vi "projekt.vi"() -> ()   [LabVIEW 2023]
doc: "Use this template to build a standard state machine design pattern. Each state executes code and determines which state to transition to. Contrast this design pattern with the User Interface Event Handler pattern, in which code executes in response to user actions. Contrast this design pattern also with the Queued Message Handler pattern, in which each message handling code can queue zero or more new messages.\nNote: This template does not contain the most recent programming guidelines recommended by National Instruments. For a complete, project-based implementation of the Standard State Machine pattern, use the Create Project dialog box instead of this template."
uses:
  projekt.ctl
  <vilib>/DAQmx/read.llb/DAQmx Read (Analog DBL 1Chan 1Samp).vi
  <vilib>/DAQmx/read.llb/DAQmx Read (Digital 1D Bool 1Chan 1Samp).vi
  <vilib>/DAQmx/write.llb/DAQmx Write (Digital 1D Bool 1Chan 1Samp).vi
  <vilib>/DAQmx/create/channels.llb/DAQmx Create Channel (AI-Voltage-Basic).vi
  <vilib>/DAQmx/create/channels.llb/DAQmx Create Channel (DI-Digital Input).vi
  <vilib>/DAQmx/create/channels.llb/DAQmx Create Channel (DO-Digital Output).vi
  <vilib>/Utility/file.llb/Read Delimited Spreadsheet (DBL).vi
  <vilib>/DAQmx/miscellaneous.llb/DAQmx Fill In Error Info.vi
  <vilib>/Utility/file.llb/Write Delimited Spreadsheet (DBL).vi
panel:
  out "TRYB":string="USTAWIENIA"
  out "wynik":i32
  out "punkty za ruch":i32=6
  out "czas wyswietlania":u32=250
  out "check index":i32
  out "now click":u32
  in  "time options":u32[](array[numeric])=[250, 500, 750, 1000, 1250, 1500]
  out "TOP WYNIKI":string="4\n4\r\n"
  out "?":string
  out "check result":bool
  in  "file path (dialog if empty)":path
  out "sekwencja":string="2\r\n"
  out "level":i32
  in  "stop":bool
  in  "Diody wynik":tag="Dev2/port0/line3:5"
  in  "Diody gorne":tag="Dev2/port0/line0:2"
  in  "Przyciski":tag="Dev2/port1/line0:2"
  in  "Pokretlo":tag="Dev2/ai1"
  # "TRYB USTAWIENIA:\nMozesz regulowac czas wyswietlania elementu sekwencji, wplywa to na liczbe punktow przyznawana za kazdy poprawny ruch.\nAby rozpoczac gre kliknij zielony guzik.\n\nTRYB GRY:\nPo wyswietleniu sekwencji na gornych diodach odwzoruj ja na guzikach.\n\nPo przegranej mozesz ponownie rozpoczac gre zielonym guzikiem!"
  # "4 green 2 yellow 1 red"
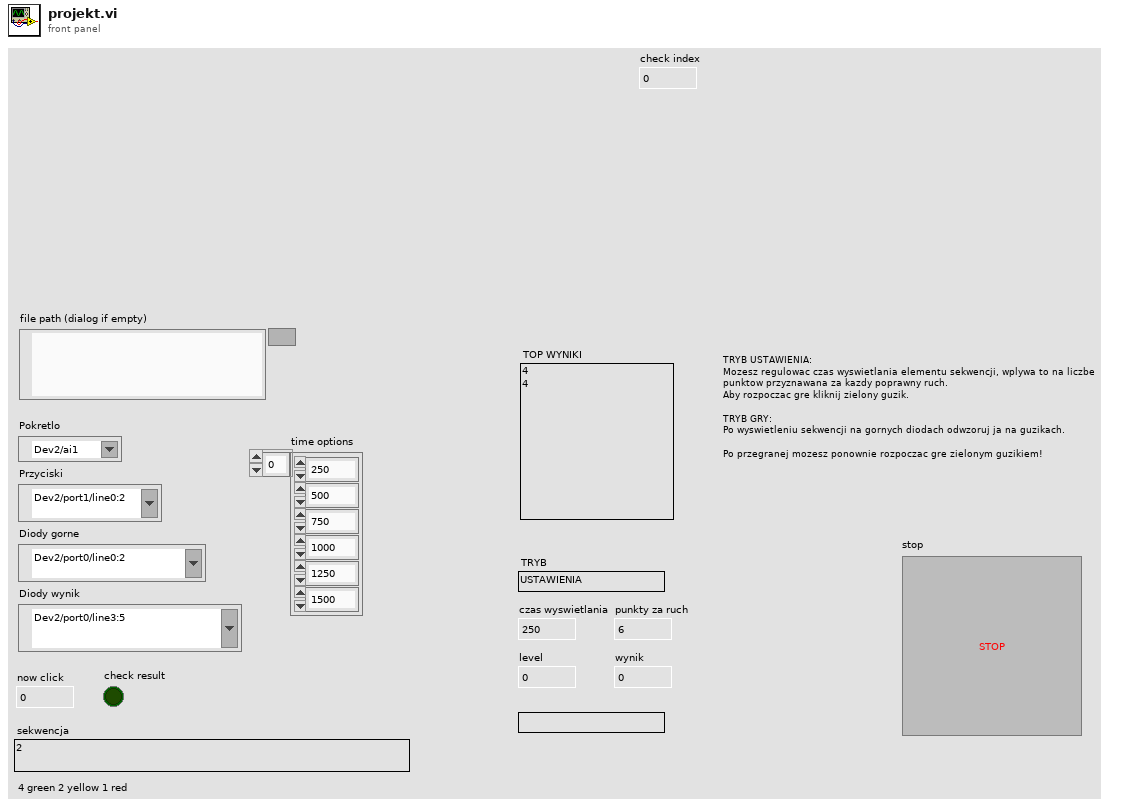
[diagram p1: front panel]
types:
  T1 = typedef "projekt.ctl" = enum16{"Initialize", "Start", "Add element", "Display ", "Check", "Game over", "Game result", "High score", "Stop"}
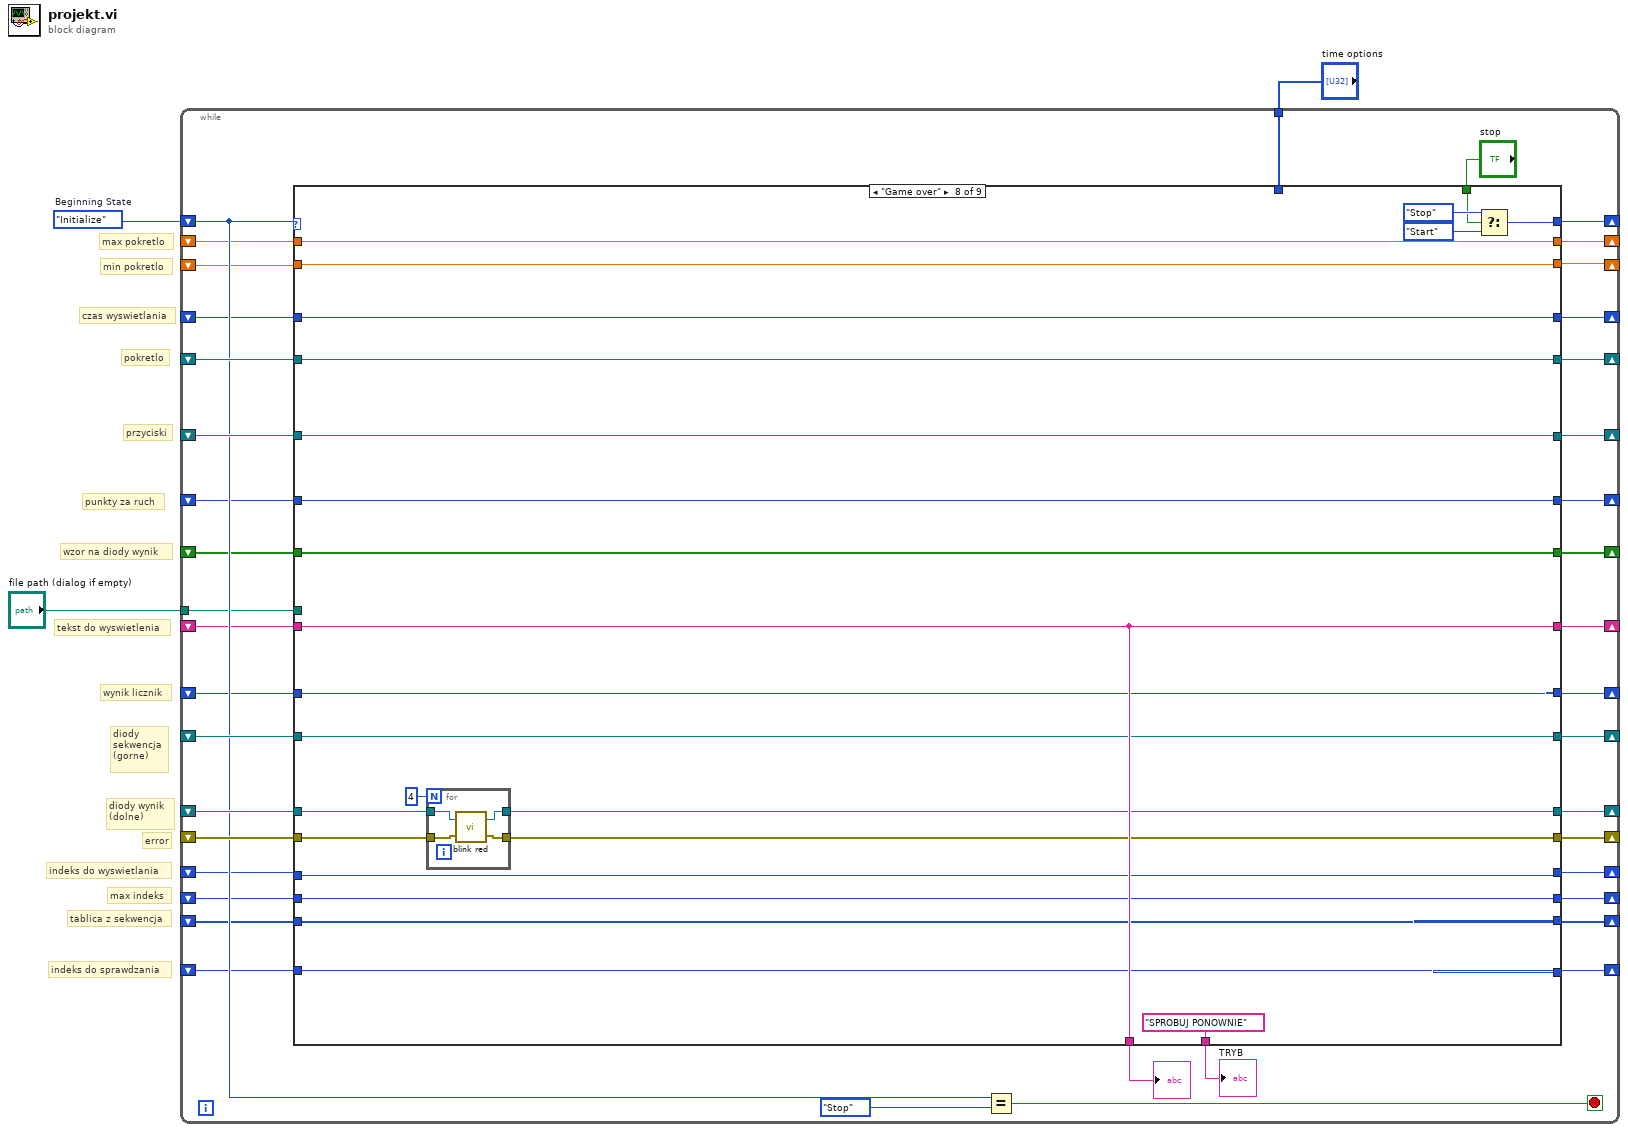
[diagram p0: block diagram]
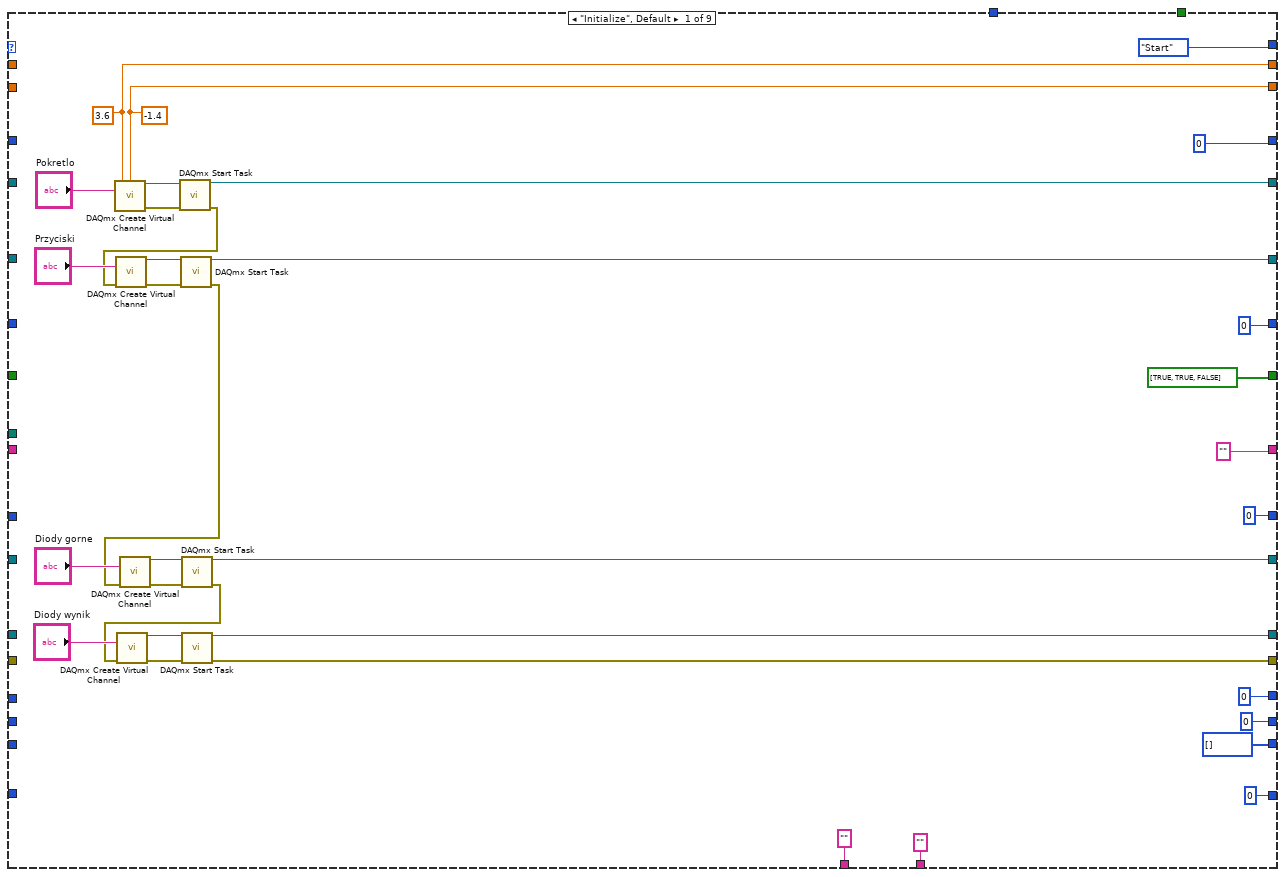
[diagram p2: hidden frame]
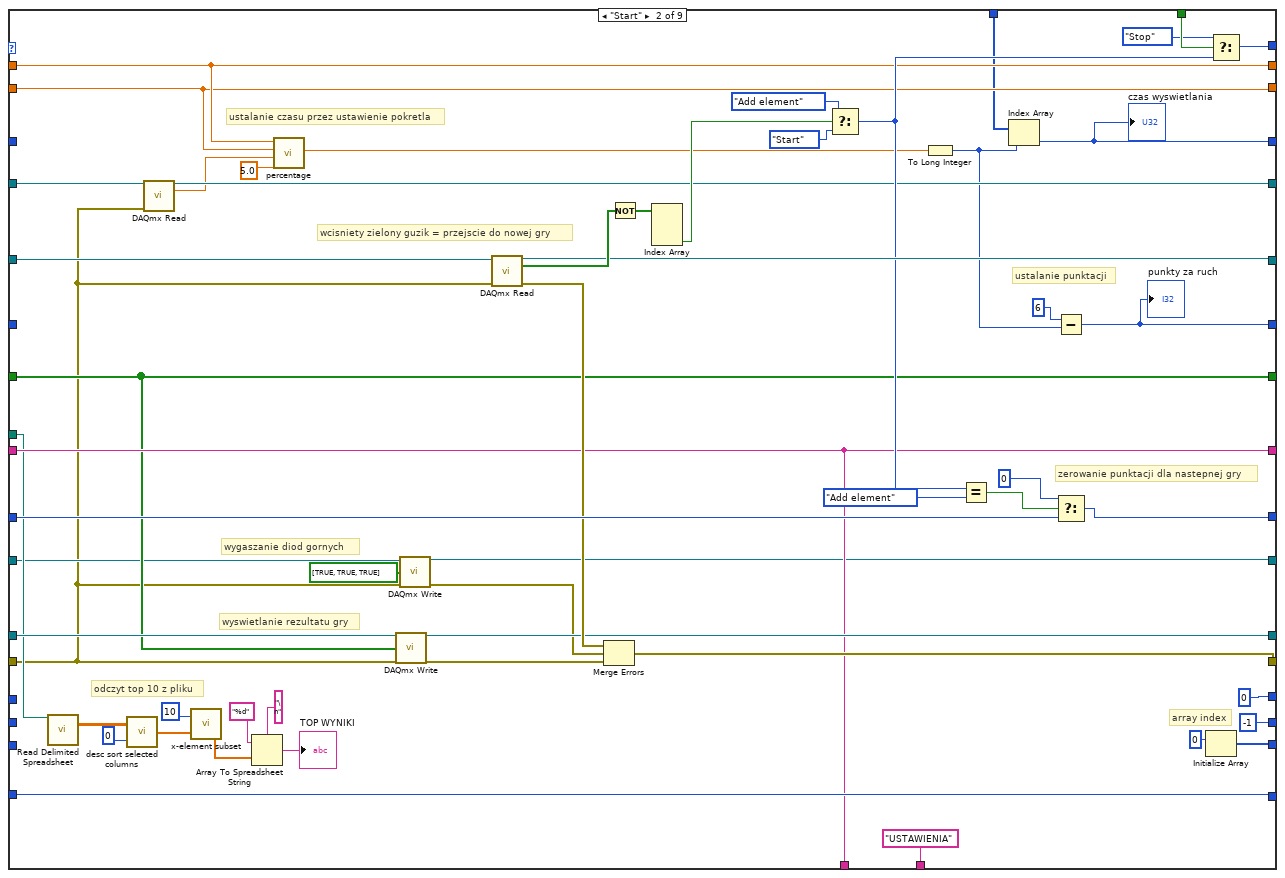
[diagram p3: hidden frame]
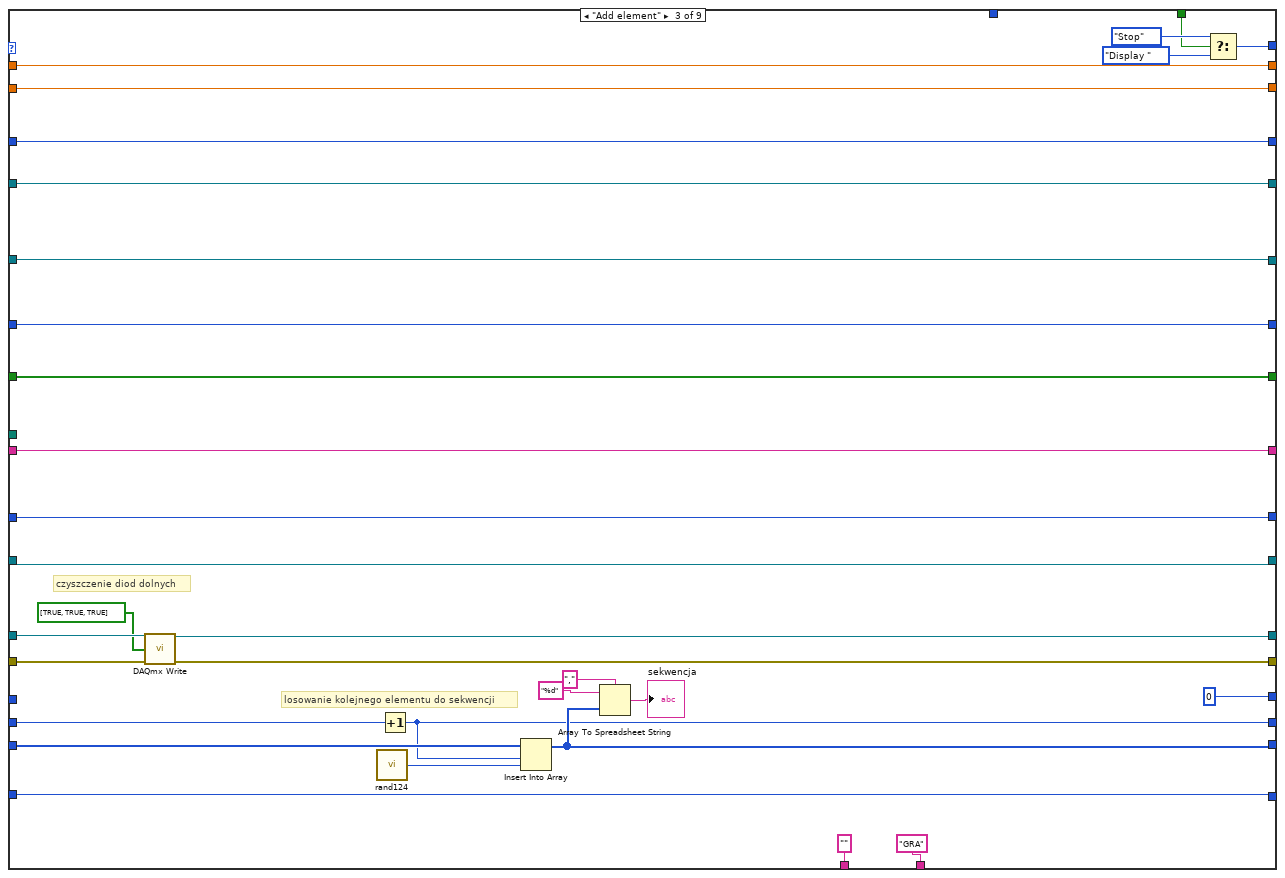
[diagram p4: hidden frame]
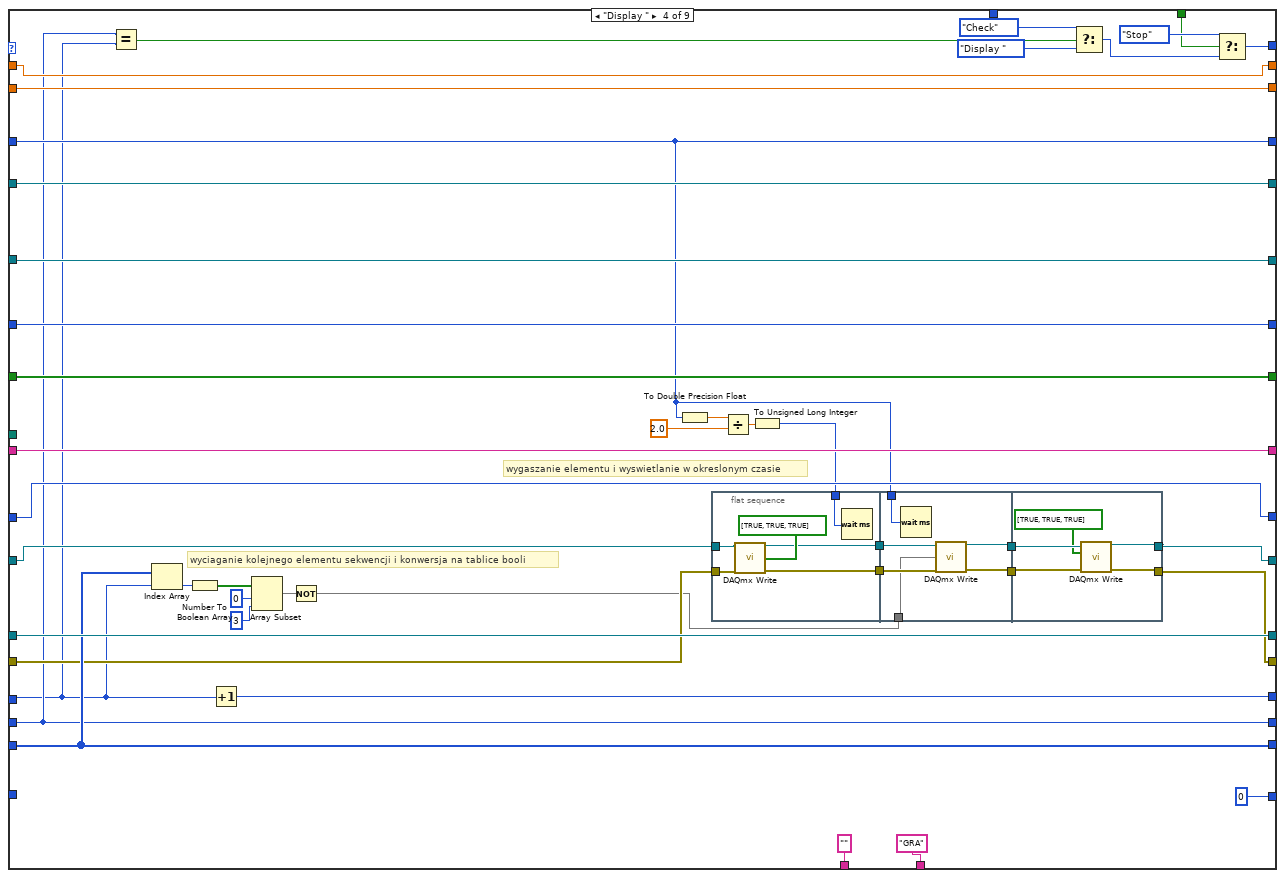
[diagram p5: hidden frame]
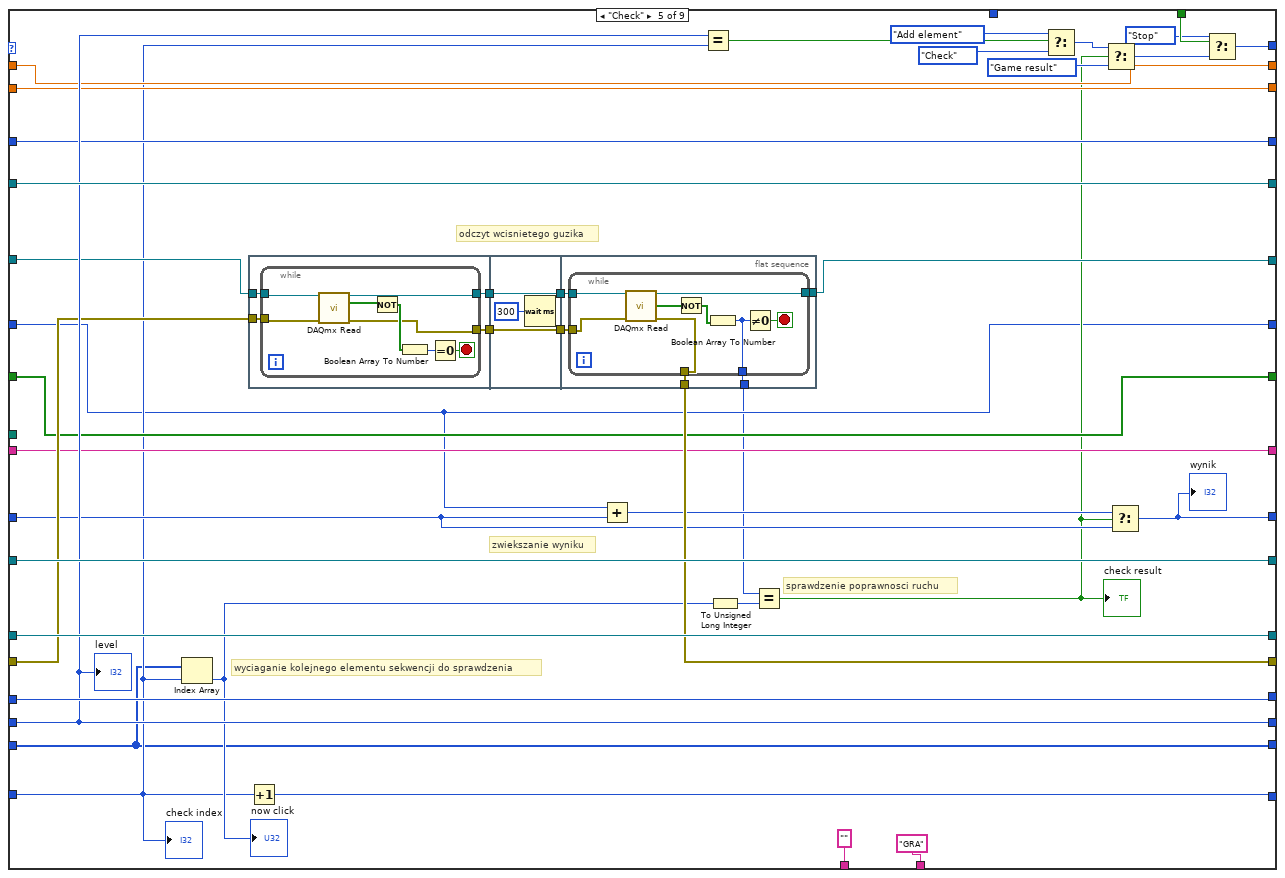
[diagram p6: hidden frame]
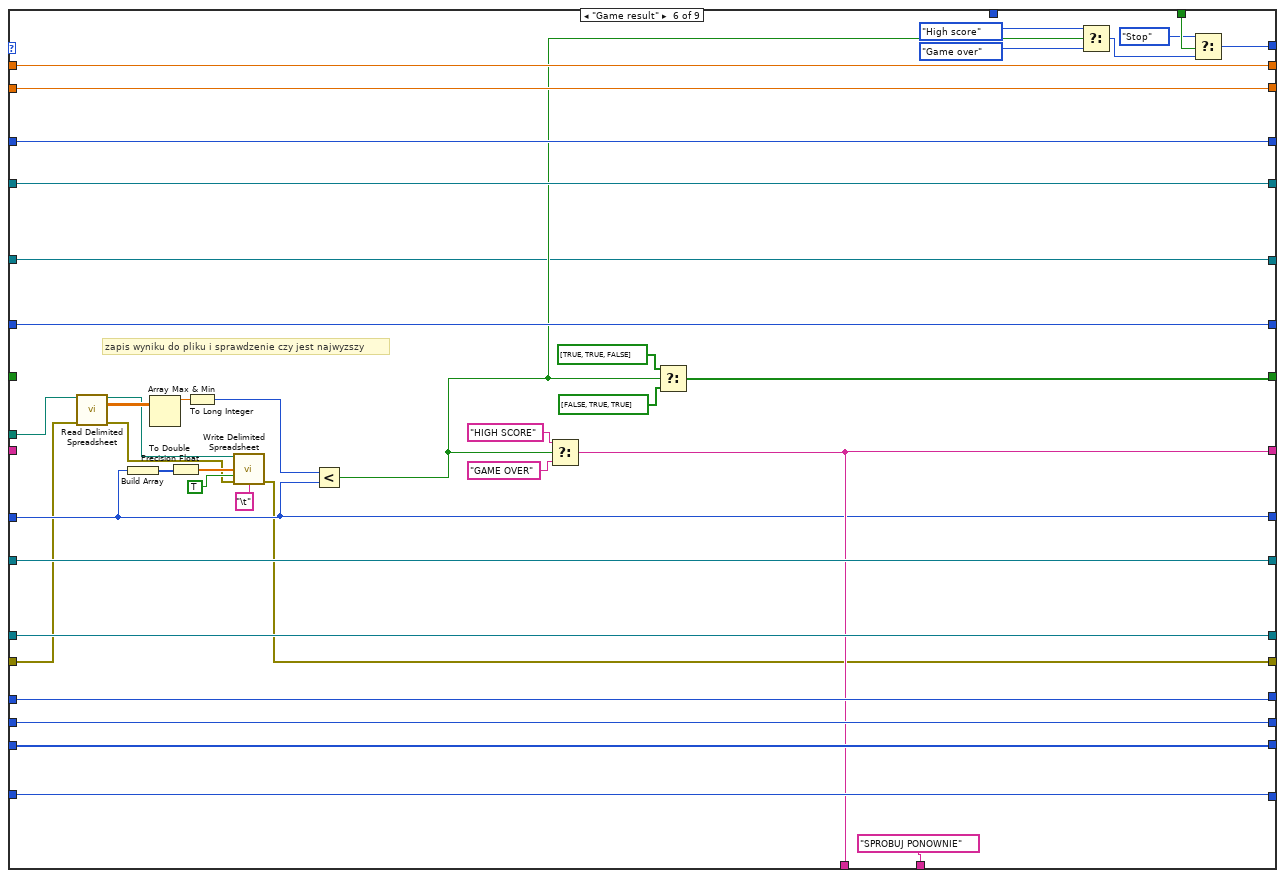
[diagram p7: hidden frame]
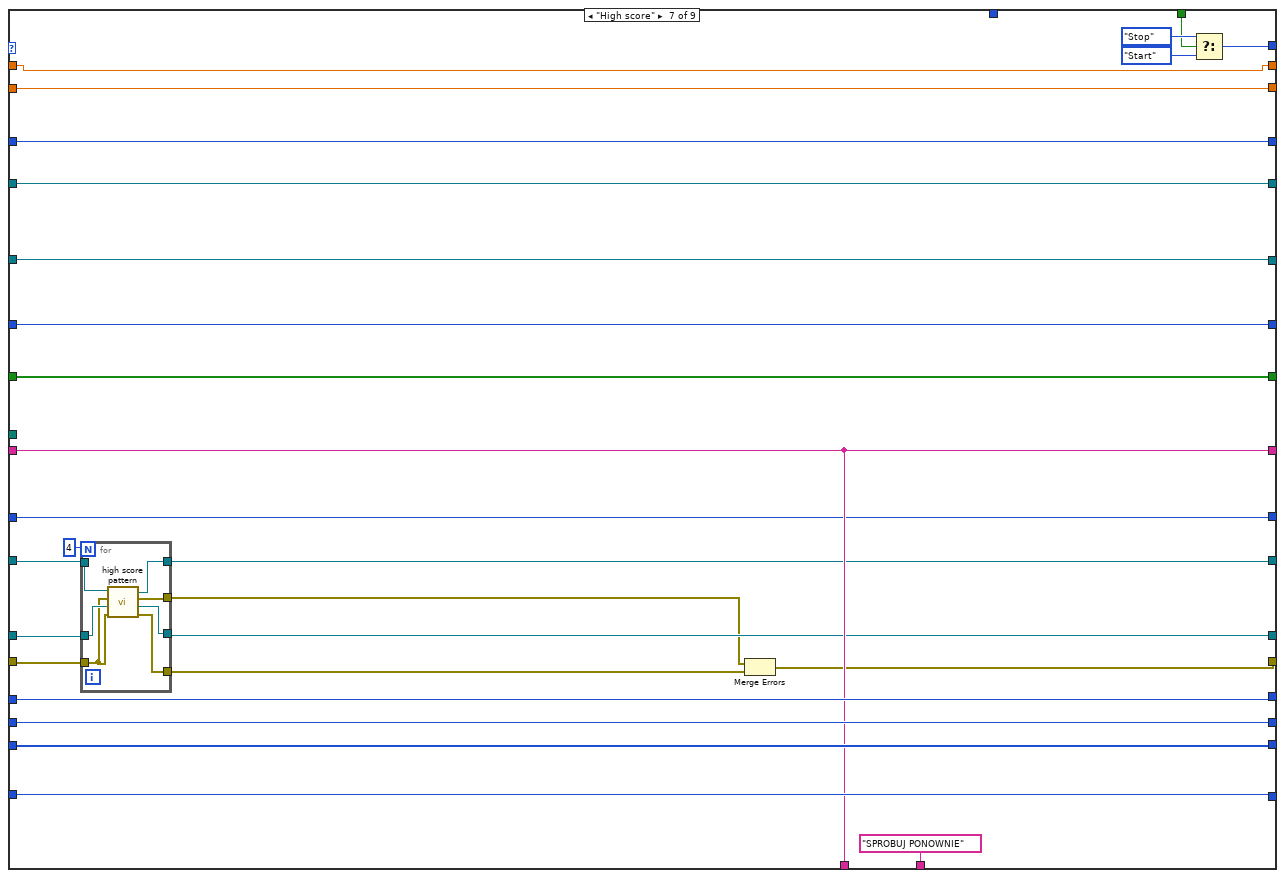
[diagram p8: hidden frame]
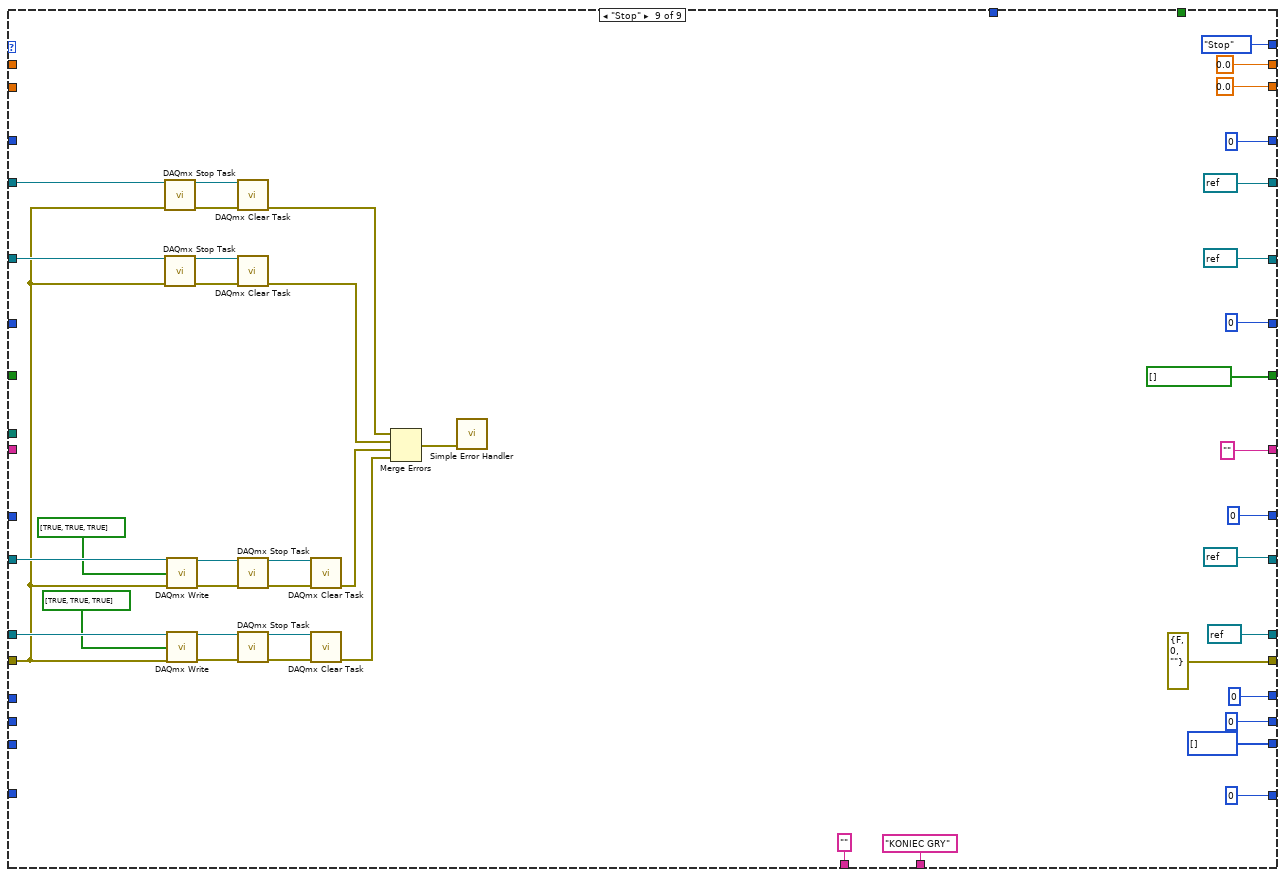
[diagram p9: hidden frame]
diagram:
  w3 = projekt."Initialize"  # Beginning State
  # "tekst do wyswietlenia"
  # "punkty za ruch"
  # "czas wyswietlania"
  # "max pokretlo"
  # "min pokretlo"
  # "wzor na diody wynik"
  # "wynik licznik"
  # "indeks do sprawdzania"
  # "tablica z sekwencja"
  # "max indeks"
  # "indeks do wyswietlania"
  # "error"
  # "diody wynik\n(dolne)"
  # "diody \nsekwencja\n(gorne)"
  # "przyciski"
  # "pokretlo"
  n1 = while {
    shift-right: [w42] -> _
    shift-left: w3 -> [w30]
    shift-right: [w34] -> _
    shift-left: _ -> [w35]
    shift-right: [w41] -> _
    shift-left: _ -> [w38]
    shift-right: [w33] -> _
    shift-left: _ -> [w39]
    shift-right: [w32] -> _
    shift-left: _ -> [w36]
    shift-right: [w40] -> _
    shift-left: _ -> [w37]
    shift-right: [w24] -> _
    shift-left: _ -> [w27]
    shift-right: [w29] -> _
    shift-left: _ -> [w28]
    shift-right: [w26] -> _
    shift-left: _ -> [w25]
    shift-right: [w23] -> _
    shift-left: _ -> [w22]
    shift-right: [w19] -> _
    shift-left: _ -> [w20]
    shift-right: [w18] -> _
    shift-left: _ -> [w17]
    shift-right: [w16] -> _
    shift-left: _ -> [w15]
    shift-right: [w14] -> _
    shift-left: _ -> [w11]
    shift-right: [w13] -> _
    shift-left: _ -> [w12]
    shift-right: [w10] -> _
    shift-left: _ -> [w9]
    tunnel: "file path (dialog if empty)" -> [w8]
    tunnel: "time options" -> [w7]
    shift-right: [w6] -> _
    shift-left: _ -> [w5]
    stop <- w44 stop-if-true
    n2 = case shown="\"Game over\"" w30 {
      tunnel: [projekt."Start" w127 w159 w199 w236 w324 w354 w385 projekt."Stop" ("Next State")] -> w42
      tunnel: [w66 w112 w146 w206 w261 w329 w335 w369 refnum<k21> refnum ("task out")] -> w41
      tunnel: [w65 w130 w163 w205 w254 w303 w349 w380 refnum<k21> refnum ("task out")] -> w40
      tunnel: w39 -> [_ w85 w162 w195 w262 w330 w337 w375 w418]
      tunnel: w38 -> [_ w115 w147 w206 w261 w329 w338 w370 w415]
      tunnel: w37 -> [_ w133 w163 w205 w256 w303 w349 w380 w428]
      tunnel: w36 -> [_ w109 w164 w204 w263 w322 w350 w381 w421]
      tunnel: w35 -> [_ w83 w145 w196 w255 w294 w339 w368 w404]
      tunnel: [w64 w113 w144 w192 w253 w295 w341 w367 errorcluster {"status"=FALSE, "code"=0, "source"=""} ("error out")] -> w34
      tunnel: [w63 w84 w162 w189 w262 w330 w333 w375 refnum<k21> refnum ("task out")] -> w33
      tunnel: [w62 w108 w164 w204 w263 w322 w350 w381 refnum<k21> refnum ("task out")] -> w32
      tunnel: "stop" -> [_ w129 w158 w200 w239 w325 w355 w386 _]
      tunnel: [u32[] [] w123 w154 w202 w225 w327 w344 w372 u32[] []] -> w24
      tunnel: w27 -> [_ _ w161 w202 w225 w327 w344 w372 _]
      tunnel: [0 -1 w139 w169 w259 w321 w345 w373 0] -> w29
      tunnel: w28 -> [_ _ w156 w169 w259 w321 w345 w373 _]
      tunnel: [0 0 0 w203 w260 w328 w346 w374 0] -> w26
      tunnel: w25 -> [_ _ _ w168 w260 w328 w346 w374 _]
      tunnel: [0 w121 w155 0 w248 w326 w343 w371 0] -> w23
      tunnel: w22 -> [_ w121 w155 _ w229 w326 w343 w371 _]
      tunnel: ["" w111 "" "" "" w311 w342 w378 ""] -> w21
      tunnel: w20 -> [_ w116 w150 w188 w232 w310 w340 w376 _]
      tunnel: [0 ("t") w117 w150 w188 w242 w310 w340 w376 0] -> w19
      tunnel: ["" w111 w148 w186 w240 w311 w342 w378 ""] -> w18
      tunnel: w17 -> [_ w111 w148 w186 w240 _ w342 w378 _]
      tunnel: [bool[] [TRUE, TRUE, FALSE] ("data") w110 w149 w187 w241 w316 w347 w377 bool[] [] ("data")] -> w16
      tunnel: w15 -> [_ w110 w149 w187 w241 _ w347 w377 _]
      tunnel: [w55 w101 w141 w184 w234 w314 w352 w383 0.0 ("minimum value")] -> w14
      tunnel: [w54 w102 w142 w185 w235 w315 w353 w384 0.0 ("maximum value")] -> w13
      tunnel: w12 -> [_ w102 w142 w185 w235 w315 w353 w384 _]
      tunnel: w11 -> [_ w101 w141 w184 w234 w314 w352 w383 _]
      tunnel: [u32 0 ("Numeric") w99 w140 w175 w233 w313 w351 w382 u32 0 ("Numeric")] -> w10
      tunnel: w9 -> [_ _ w140 w175 w233 w313 w351 w382 _]
      tunnel: w8 -> [_ w107 _ _ _ w300 _ _ _]
      tunnel: w7 -> [_ w98 _ _ _ _ _ _ _]
      tunnel: [0 w90 w137 w179 w227 w312 w348 w379 0] -> w6
      tunnel: w5 -> [_ _ w137 w179 w227 w312 w348 w379 _]
      tunnel: ["" "USTAWIENIA" "GRA" "GRA" "GRA" "SPROBUJ PONOWNIE" "SPROBUJ PONOWNIE" "SPROBUJ PONOWNIE" "KONIEC GRY"] -> w4
      frame "Initialize", Default {
        w54 = 3.6 ("maximum value")
        w55 = -1.4 ("minimum value")
        n3 = call-poly <vilib>:"DAQmx Create Virtual Channel.vi"("maximum value"=w54, "minimum value"=w55, "physical channels"="Pokretlo") -> ("task out"=w73:refnum<k21>, "error out"=w74:errorcluster)  [unwired: 11 in]
        n4 = call <vilib>:"DAQmx Start Task.vi"("task/channels in"=w73, "error in"=w74) -> ("task out"=w62:refnum<k21>, "error out"=w53:errorcluster)  [unwired: 12 in]
        n5 = call-poly <vilib>:"DAQmx Create Virtual Channel.vi"("lines"="Przyciski", "error in"=w53) -> ("task out"=w60:refnum<k21>, "error out"=w59:errorcluster)  [unwired: 12 in]
        n6 = call <vilib>:"DAQmx Start Task.vi"("task/channels in"=w60, "error in"=w59) -> ("task out"=w65:refnum<k21>, "error out"=w68:errorcluster)  [unwired: 12 in]
        n7 = call-poly <vilib>:"DAQmx Create Virtual Channel.vi"("lines"="Diody gorne", "error in"=w68) -> ("task out"=w72:refnum<k21>, "error out"=w71:errorcluster)  [unwired: 12 in]
        n8 = call <vilib>:"DAQmx Start Task.vi"("task/channels in"=w72, "error in"=w71) -> ("task out"=w63:refnum<k21>, "error out"=w67:errorcluster)  [unwired: 12 in]
        n9 = call-poly <vilib>:"DAQmx Create Virtual Channel.vi"("lines"="Diody wynik", "error in"=w67) -> ("task out"=w70:refnum<k21>, "error out"=w69:errorcluster)  [unwired: 12 in]
        n10 = call <vilib>:"DAQmx Start Task.vi"("task/channels in"=w70, "error in"=w69) -> ("task out"=w66:refnum<k21>, "error out"=w64:errorcluster)  [unwired: 12 in]
      }
      frame "Start" {
        # "zerowanie punktacji dla nastepnej gry"
        # "wyswietlanie rezultatu gry"
        # "wygaszanie diod gornych"
        # "ustalanie punktacji"
        # "wcisniety zielony guzik = przejscie do nowej gry"
        # "ustalanie czasu przez ustawienie pokretla"
        # "odczyt top 10 z pliku"
        # "array index"
        n11 = call-poly <vilib>:"Read Delimited Spreadsheet.vi"("file path (dialog if empty)"=w107) -> ("all rows"=w96:dbl[][])  [unwired: 9 in, 5 out]
        n12 = call "desc sort selected columns.vi"("disabled index (col)"=0, "all rows in"=w96) -> ("1d sorted array (desc)"=w94:dbl[])
        n13 = call-poly <vilib>:"DAQmx Read.vi"("task/channels in"=w109, "error in"=w83) -> ("task out"=w108:refnum<k21>, "data"=w103:dbl)  [unwired: 11 in, 1 out]
        n14 = call "x-element subset.vi"("input array"=w94, "x elements"=10 ("y")) -> ("array subset"=w93:dbl[])
        n15 = Array To Spreadsheet String(delimiter (Tab)="\n", array=w93, 3:"%d" ("format string")) -> (spreadsheet string=→"TOP WYNIKI":string)
        n16 = call "percentage.vi"("max range"=5.0, "data read"=w103, "minimum value"=w101, "maximum value"=w102) -> ("percentage of mac range"=w91:dbl)
        n17 = call-poly <vilib>:"DAQmx Write.vi"("task/channels in"=w115, "data"=w110, "error in"=w83) -> ("task out"=w112:refnum<k21>, "error out"=w82:errorcluster)  [unwired: 10 in, 1 out]
        n18 = call-poly <vilib>:"DAQmx Write.vi"("task/channels in"=w85, "data"=bool[] [TRUE, TRUE, TRUE], "error in"=w83) -> ("task out"=w84:refnum<k21>, "error out"=w81:errorcluster)  [unwired: 10 in, 1 out]
        n19 = call-poly <vilib>:"DAQmx Read.vi"("task/channels in"=w133, "error in"=w83) -> ("task out"=w130:refnum<k21>, "data"=w131:bool[], "error out"=w114:errorcluster)  [unwired: 11 in]
        n20 = Merge Errors(w114, w81, w82) -> (w113:errorcluster)
        n21 = Not(x=w131) -> (.not. x?=w132:bool[])
        n22 = Index Array(array=w132) -> (element #3=w126:bool)  [unwired: 3 in, 2 out]
        n23 = Select(t=projekt."Add element" ("Next State"), s=w126, f=projekt."Start" ("Next State")) -> (s? t:f=w120:T1)
        n24 = To Long Integer(number=w91) -> (32bit integer=w89:i32)
        n25 = Equal?(x=w120, y=projekt."Add element") -> (x = y?=w118:bool)
        n26 = Index Array(array=w98, index=w89) -> (element=w99:u32)
        "czas wyswietlania" <- w99
        n27 = Subtract(x=6, y=w89) -> (x-y=w90:i32)
        "punkty za ruch" <- w90
        n28 = Select(t=0, s=w118, f=w116) -> (s? t:f=w117:i32)
        n29 = Initialize Array(u32 0 ("element")) -> (w123:u32[])  [unwired: 1 in]
        n30 = Select(t=projekt."Stop" ("Next State"), s=w129, f=w120) -> (s? t:f=w127:T1)
      }
      frame "Add element" {
        # "losowanie kolejnego elementu do sekwencji"
        # "czyszczenie diod dolnych"
        n31 = call-poly <vilib>:"DAQmx Write.vi"("task/channels in"=w147, "data"=bool[] [TRUE, TRUE, TRUE], "error in"=w145) -> ("task out"=w146:refnum<k21>, "error out"=w144:errorcluster)  [unwired: 10 in, 1 out]
        n32 = call "rand124.vi"() -> ("rand"=w138:u32)
        n33 = Increment(x=w156) -> (x+1=w139:i32)
        n34 = Insert Into Array(array=w161, index=w139, new element=w138) -> (w154:u32[])
        n35 = Array To Spreadsheet String(delimiter (Tab)=",", array=w154, 3:"%d" ("format string")) -> (spreadsheet string=→"sekwencja":string)
        n36 = Select(t=projekt."Stop" ("Next State"), s=w158, f=projekt."Display " ("Next State")) -> (s? t:f=w159:T1)
      }
      frame "Display " {
        # "wygaszanie elementu i wyswietlanie w okreslonym czasie"
        # "wyciaganie kolejnego elementu sekwencji i konwersja na tablice booli"
        n37 = Equal?(x=w169, y=w168) -> (x = y?=w167:bool)
        n38 = Index Array(array=w202, index=w168) -> (element=w183:u32)
        n39 = Number To Boolean Array(number=w183) -> (Boolean array=w182:bool[])
        n40 = Increment(x=w168) -> (x+1=w203:i32)
        n41 = Array Subset(array=w182, index=0, length=3) -> (w177:bool[])
        n42 = Not(x=w177) -> (.not. x?=w176:bool[])
        n43 = To Double Precision Float(number=w175) -> (double precision float=w174:dbl)
        n44 = flat-sequence {
          tunnel: w195 -> [w212]
          tunnel: w196 -> [w211]
          tunnel: [w209] -> w194
          tunnel: [w208] -> w193
          tunnel: w171 -> [w207]
          tunnel: w194 -> [w217]
          tunnel: w193 -> [w216]
          tunnel: [w218] -> w191
          tunnel: [w215] -> w190
          tunnel: w175 -> [w214]
          tunnel: w176 -> [w213]
          tunnel: [w222] -> w189
          tunnel: [w220] -> w192
          tunnel: w191 -> [w221]
          tunnel: w190 -> [w223]
          frame #0 {
            n45 = call-poly <vilib>:"DAQmx Write.vi"("task/channels in"=w212, "data"=bool[] [TRUE, TRUE, TRUE], "error in"=w211) -> ("task out"=w208:refnum<k21>, "error out"=w209:errorcluster)  [unwired: 10 in, 1 out]
            n46 = Wait (ms)(milliseconds to wait=w207) -> ()  [unwired: 1 out]
          }
          frame #1 {
            n47 = Wait (ms)(milliseconds to wait=w214) -> ()  [unwired: 1 out]
            n48 = call-poly <vilib>:"DAQmx Write.vi"("task/channels in"=w216, "data"=w213, "error in"=w217) -> ("task out"=w215:refnum<k21>, "error out"=w218:errorcluster)  [unwired: 10 in, 1 out]
          }
          frame #2 {
            n49 = call-poly <vilib>:"DAQmx Write.vi"("task/channels in"=w223, "data"=bool[] [TRUE, TRUE, TRUE], "error in"=w221) -> ("task out"=w222:refnum<k21>, "error out"=w220:errorcluster)  [unwired: 10 in, 1 out]
          }
        }
        n50 = Divide(x=w174, y=2.0) -> (x/y=w172:dbl)
        n51 = To Unsigned Long Integer(number=w172) -> (unsigned 32bit integer=w171:u32)
        n52 = Select(t=projekt."Check" ("Next State"), s=w167, f=projekt."Display " ("Next State")) -> (s? t:f=w197:T1)
        n53 = Select(t=projekt."Stop" ("Next State"), s=w200, f=w197) -> (s? t:f=w199:T1)
      }
      frame "Check" {
        # "sprawdzenie poprawnosci ruchu"
        # "odczyt wcisnietego guzika"
        # "wyciaganie kolejnego elementu sekwencji do sprawdzenia"
        # "zwiekszanie wyniku"
        n54 = Index Array(array=w225, index=w229) -> (element=w244:u32)
        "now click" <- w244
        n55 = flat-sequence {
          tunnel: w256 -> [w267]
          tunnel: w255 -> [w266]
          tunnel: [w265] -> w252
          tunnel: [w264] -> w250
          tunnel: w252 -> [w278]
          tunnel: [w278] -> w251
          tunnel: w250 -> [w277]
          tunnel: [w277] -> w249
          tunnel: w251 -> [w283]
          tunnel: w249 -> [w282]
          tunnel: [w281] -> w254
          tunnel: [w280] -> w253
          tunnel: [w279] -> w226
          frame #0 {
            n56 = while {
              tunnel: w267 -> [w273]
              tunnel: w266 -> [w272]
              tunnel: [w271] -> w265
              tunnel: [w270] -> w264
              stop <- w268 stop-if-true
              n57 = call-poly <vilib>:"DAQmx Read.vi"("task/channels in"=w273, "error in"=w272) -> ("task out"=w271:refnum<k21>, "data"=w274:bool[], "error out"=w270:errorcluster)  [unwired: 11 in]
              n58 = Not(x=w274) -> (.not. x?=w275:bool[])
              n59 = Boolean Array To Number(Boolean array=w275) -> (number=w269:u32)
              n60 = Equal To 0?(x=w269) -> (x = 0?=w268:bool)
            }
          }
          frame #1 {
            n61 = Wait (ms)(milliseconds to wait=u32 300) -> ()  [unwired: 1 out]
          }
          frame #2 {
            n62 = while {
              tunnel: w283 -> [w290]
              tunnel: w282 -> [w289]
              tunnel: [w287] -> w281
              tunnel: [w286] -> w280
              tunnel: [w284] -> w279
              stop <- w285 stop-if-true
              n63 = call-poly <vilib>:"DAQmx Read.vi"("task/channels in"=w290, "error in"=w289) -> ("task out"=w287:refnum<k21>, "data"=w288:bool[], "error out"=w286:errorcluster)  [unwired: 11 in]
              n64 = Not(x=w288) -> (.not. x?=w291:bool[])
              n65 = Boolean Array To Number(Boolean array=w291) -> (number=w284:u32)
              n66 = Not Equal To 0?(x=w284) -> (x != 0?=w285:bool)
            }
          }
        }
        n67 = Increment(x=w229) -> (x+1=w248:i32)
        n68 = Add(x=w227, y=w232) -> (x+y=w231:i32)
        n69 = Equal?(x=w259, y=w229) -> (x = y?=w258:bool)
        n70 = To Unsigned Long Integer(number=w244) -> (unsigned 32bit integer=w245:u32)
        n71 = Equal?(x=w226, y=w245) -> (x = y?=w228:bool)
        "check result" <- w228
        n72 = Select(t=projekt."Add element" ("States"), s=w258, f=projekt."Check" ("States")) -> (s? t:f=w247:T1)
        n73 = Select(t=w247, s=w228, f=projekt."Game result" ("States")) -> (s? t:f=w238:T1)
        n74 = Select(t=w231, s=w228, f=w232) -> (s? t:f=w242:i32)
        "wynik" <- w242
        n75 = Select(t=projekt."Stop", s=w239, f=w238) -> (s? t:f=w236:T1)
        "level" <- w259
        "check index" <- w229
      }
      frame "Game result" {
        # "zapis wyniku do pliku i sprawdzenie czy jest najwyzszy"
        n76 = call-poly <vilib>:"Read Delimited Spreadsheet.vi"("file path (dialog if empty)"=w300, "error in (no error)"=w294) -> ("new file path (Not A Path if cancelled)"=w298:path, "all rows"=w302:dbl[][], "error out"=w293:errorcluster)  [unwired: 8 in, 3 out]
        n77 = Build Array(w310) -> (w309:i32[])
        n78 = Array Max & Min(array=w302) -> (max value=w301:dbl)  [unwired: 3 out]
        n79 = To Double Precision Float(number=w309) -> (double precision float=w308:dbl[])
        n80 = To Long Integer(number=w301) -> (32bit integer=w299:i32)
        n81 = call-poly <vilib>:"Write Delimited Spreadsheet.vi"("file path (dialog if empty)"=w298, "1D data"=w308, "append to file? (new file:F)"=TRUE, "error in (no error)"=w293, "delimiter (\\t)"="\t" ("delimiter (\\t)")) -> ("error out"=w295:errorcluster)  [unwired: 9 in, 1 out]
        n82 = Less?(x=w299, y=w310) -> (x < y?=w305:bool)
        n83 = Select(t="HIGH SCORE", s=w305, f="GAME OVER") -> (s? t:f=w311:string)
        n84 = Select(t=bool[] [TRUE, TRUE, FALSE] ("data"), s=w305, f=bool[] [FALSE, TRUE, TRUE] ("data")) -> (s? t:f=w316:bool[])
        n85 = Select(t=projekt."High score" ("States"), s=w305, f=projekt."Game over" ("States")) -> (s? t:f=w307:T1)
        n86 = Select(t=projekt."Stop" ("States"), s=w325, f=w307) -> (s? t:f=w324:T1)
      }
      frame "High score" {
        n87 = for {
          N: 4 -> [_]
          tunnel: w339 -> [w363]
          tunnel: w338 -> [w364]
          tunnel: w337 -> [w362]
          tunnel: [w361] -> w336
          tunnel: [w360] -> w335
          tunnel: [w359] -> w334
          tunnel: [w358] -> w333
          n88 = call "high score pattern.vi"("error in \n(diody gora)"=w363, "task in\n(diody dol)"=w364, "error in\n(diody dol)"=w363, "task in \n(diody gora)"=w362) -> ("error out\n(diody dolne)"=w361:errorcluster, "task out\n(diody dolne)"=w360:refnum<k21>, "error out\n(diody gorne)"=w359:errorcluster, "task out\n(diody gorne)"=w358:refnum<k21>)
        }
        n89 = Merge Errors(w334, w336) -> (w341:errorcluster)
        n90 = Select(t=projekt."Stop" ("States"), s=w355, f=projekt."Start" ("States")) -> (s? t:f=w354:T1)
      }
      frame "Game over" {
        n91 = for {
          N: 4 -> [_]
          tunnel: w370 -> [w390]
          tunnel: [w392] -> w369
          tunnel: w368 -> [w389]
          tunnel: [w391] -> w367
          n92 = call "blink red.vi"("error in"=w389, "task in\n(diody dolne)"=w390) -> ("error out"=w391:errorcluster, "task out\n(diody dolne)"=w392:refnum<k21>)
        }
        n93 = Select(t=projekt."Stop" ("States"), s=w386, f=projekt."Start" ("States")) -> (s? t:f=w385:T1)
      }
      frame "Stop" {
        n94 = call <vilib>:"DAQmx Stop Task.vi"("task/channels in"=w421, "error in"=w404) -> ("task out"=w427:refnum<k21>, "error out"=w426:errorcluster)  [unwired: 12 in]
        n95 = call <vilib>:"DAQmx Stop Task.vi"("task/channels in"=w428, "error in"=w404) -> ("task out"=w430:refnum<k21>, "error out"=w429:errorcluster)  [unwired: 12 in]
        n96 = call-poly <vilib>:"DAQmx Write.vi"("task/channels in"=w418, "data"=bool[] [TRUE, TRUE, TRUE], "error in"=w404) -> ("task out"=w419:refnum<k21>, "error out"=w416:errorcluster)  [unwired: 10 in, 1 out]
        n97 = call-poly <vilib>:"DAQmx Write.vi"("task/channels in"=w415, "data"=bool[] [TRUE, TRUE, TRUE], "error in"=w404) -> ("task out"=w413:refnum<k21>, "error out"=w414:errorcluster)  [unwired: 10 in, 1 out]
        n98 = call <vilib>:"DAQmx Clear Task.vi"("task in"=w427, "error in"=w426) -> ("error out"=w403:errorcluster)  [unwired: 13 in]
        n99 = call <vilib>:"DAQmx Clear Task.vi"("task in"=w430, "error in"=w429) -> ("error out"=w425:errorcluster)  [unwired: 13 in]
        n100 = call <vilib>:"DAQmx Stop Task.vi"("task/channels in"=w419, "error in"=w416) -> ("task out"=w434:refnum<k21>, "error out"=w433:errorcluster)  [unwired: 12 in]
        n101 = call <vilib>:"DAQmx Stop Task.vi"("task/channels in"=w413, "error in"=w414) -> ("task out"=w432:refnum<k21>, "error out"=w431:errorcluster)  [unwired: 12 in]
        n102 = call <vilib>:"DAQmx Clear Task.vi"("task in"=w434, "error in"=w433) -> ("error out"=w424:errorcluster)  [unwired: 13 in]
        n103 = call <vilib>:"DAQmx Clear Task.vi"("task in"=w432, "error in"=w431) -> ("error out"=w423:errorcluster)  [unwired: 13 in]
        n104 = Merge Errors(w403, w425, w424, w423) -> (w422:errorcluster)
        n105 = call <vilib>:"Simple Error Handler.vi"("error in (no error)"=w422) -> ()  [unwired: 4 in, 5 out]
      }
    }
    "?" <- w21
    "TRYB" <- w4
    n106 = Equal?(x=w30, y=projekt."Stop" ("States")) -> (x = y?=w44:bool)
  }
